vi "GSCS_Server.vi"   [LabVIEW 2015]
uses:
  Users/Sherman/Desktop/BETA_GSCS/Systems/SystemUtil/Command.ctl
  Users/Sherman/Desktop/BETA_GSCS/Log/LogItem.ctl
  Users/Sherman/Desktop/BETA_GSCS/Systems/TCPServer/TCPServer_Global.vi
types:
  T1 = typedef "Command.ctl" = cluster{"Command":string, "Parameter":string}
  T2 = typedef "LogItem.ctl" = cluster{"error in (no error)":errorcluster, "Source":string, "Comment ":string}
  T3 = enum16{"Launch", "Log", "Open", "Close", "Shutdown"}
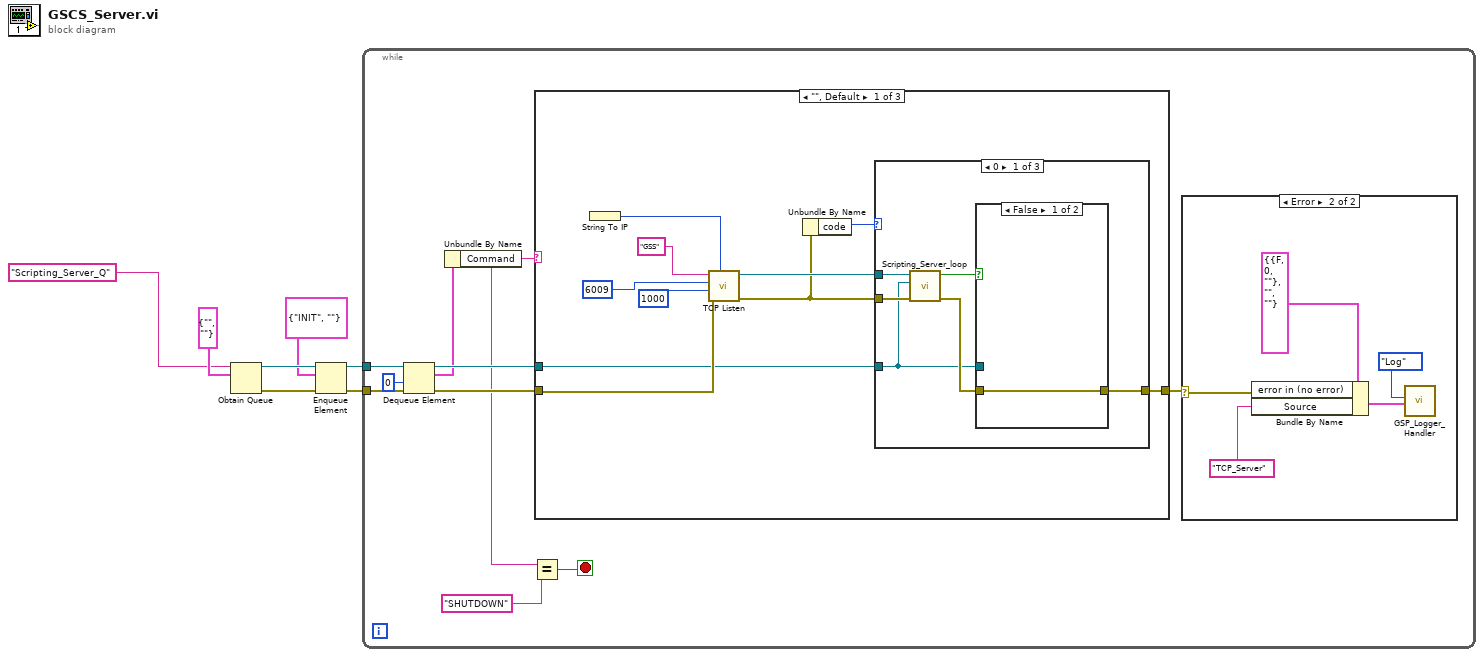
[diagram p0: block diagram]
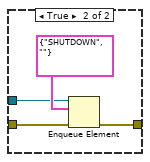
[diagram p3: hidden frame]
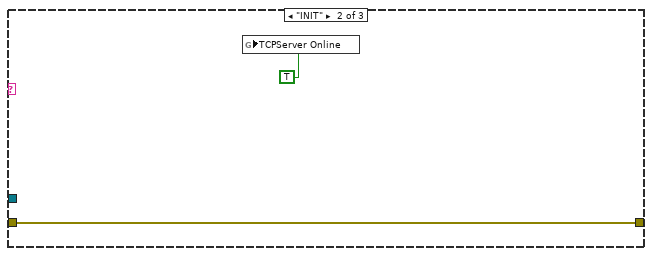
[diagram p6: hidden frame]
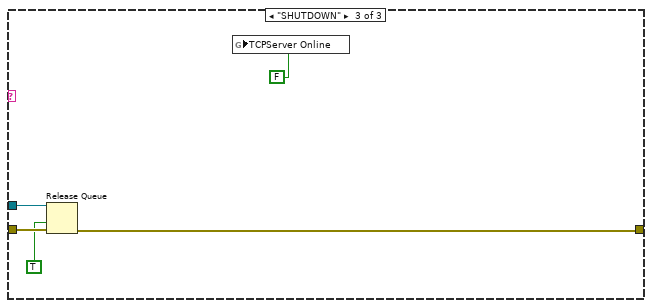
[diagram p7: hidden frame]
diagram:
  n1 = Obtain Queue(name (unnamed)="Scripting_Server_Q", element data type=T1 {"Command"="", "Parameter"=""} ("Command")) -> (queue out=w4:refnum<queue>, error out=w3:errorcluster)  [unwired: 3 in, 1 out]
  n2 = Enqueue Element(queue=w4, element=T1 {"Command"="INIT", "Parameter"=""}, error in (no error)=w3) -> (queue out=w6:refnum<queue>, error out=w5:errorcluster)  [unwired: 1 in, 1 out]
  n3 = while {
    tunnel: w6 -> [w17]
    tunnel: w5 -> [w16]
    stop <- w9 stop-if-true
    n4 = Dequeue Element(queue=w17, timeout in ms (-1)=0, error in (no error)=w16) -> (queue out=w15:refnum<queue>, element=w13:T1, error out=w14:errorcluster)  [unwired: 1 out]
    n5 = Unbundle By Name(w13) -> ("Command"=w11:string)
    n6 = Equal?(x=w11, y="SHUTDOWN") -> (x = y?=w9:bool)
    n7 = case shown="\"\", Default" w11 {
      tunnel: w15 -> [w29 _ w50]
      tunnel: w14 -> [w30 w44 w49]
      tunnel: [w28 w44 w47] -> w8
      frame "", Default {
        n8 = String To IP() -> (0:w25:u32)  [unwired: 1 in]
        n9 = call <vilib>:"TCP Listen.vi"("net address"=w25, "error in (no error)"=w30, "timeout ms (wait forever: -1)"=1000, "port"=6009 ("timeout ms (wait forever: -1)"), "service name"="GSS") -> ("error out"=w26:errorcluster, "connection ID"=w27:refnum<k5>)  [unwired: 2 in, 3 out]
        n10 = Unbundle By Name(w26) -> ("code"=w32:i32)
        n11 = case shown="0" w32 {
          tunnel: w27 -> [w38 _ _]
          tunnel: w26 -> [w37 _ _]
          tunnel: w29 -> [w33 _ _]
          tunnel: [w34 _ _] -> w28
          frame 0 {
            n12 = call "Scripting_Server_loop.vi"("error in (no error)"=w37, "queue in"=w33, "TCP Connection ID"=w38) -> ("error out"=w35:errorcluster, "Shutdown?"=w36:bool)  [unwired: 3 in]
            n13 = case shown="False" w36 {
              tunnel: w35 -> [w39 w43]
              tunnel: [w39 w42] -> w34
              tunnel: w33 -> [_ w40]
              frame False {
              }
              frame True {
                n14 = Enqueue Element(queue=w40, element=T1 {"Command"="SHUTDOWN", "Parameter"=""}, error in (no error)=w43) -> (error out=w42:errorcluster)  [unwired: 1 in, 2 out]
              }
            }
          }
          frame 1, Default {
          }
          frame 56 {
          }
        }
      }
      frame "INIT" {
        n15 = global write "TCPServer_Global.vi" "TCPServer Online"(TRUE) -> ()
      }
      frame "SHUTDOWN" {
        n16 = Release Queue(queue=w50, force destroy? (F)=TRUE, error in (no error)=w49) -> (error out=w47:errorcluster)  [unwired: 2 out]
        n17 = global write "TCPServer_Global.vi" "TCPServer Online"(FALSE) -> ()
      }
    }
    n18 = case shown="Error" w8 {
      selector: w8 -> [_ w18]
      frame No Error {
      }
      frame Error {
        n19 = Bundle By Name(cluster=T2 {"error in (no error)"={"status"=FALSE, "code"=0, "source"=""}, "Source"="", "Comment "=""} ("Log"), "error in (no error)"=w18, "Source"="TCP_Server") -> (w21:T2)
        n20 = call "GSP_Logger_Handler.vi"("Log"=w21, "Actions"=T3."Log") -> ()  [unwired: 5 in, 1 out]
      }
    }
  }
